vi "SerialCharWriteReadnoopen.vi"(0 "VISA resource name":refnum<visa-resource-name>, 3 "write buffer":string) -> (10 "read buffer":string)   [LabVIEW 2012]
doc: "The Basic Serial Read and Write example performs a Serial Port Read, a Serial Port Write, or a combination of these actions. The user selects the actions (read or write) on the front panel. If both are selected, the VI will write the data first, read data, and then close the VISA session that is opened to the port. This VI will wait until the specified number of bytes is received at the port. Only the number of bytes specified will be read.\n\nINSTRUCTIONS:\n1) Select the serial resource and configuration parameters (baud rate, data bits, parity, stop bits, flow control).\n2) Select the operations to be performed. \n3) Connect the serial port to your device. If no device is available, perform a loopback test by doing one of the following. Short pins 2 and 3 on a RS-232 cable or short pin 4 to pin 8 and pin 5 to pin 9 on a RS-485/422 cable. \n4) Run the VI to see the data read. (The \"read string\" will match the \"string to write\" if a loopback test was performed.)\n\nNote: The parameters set for the serial port must match the parameters of the connected instrument or device. In this example, the bytes to read parameter specifies the number of bytes that the serial port reads. If there were more bytes at the port than the number specified in bytes to read, those bytes would not be read. Also, if you specify to read more bytes than the number of bytes actually read, you might receive a timeout error message.\n\nOn the block diagram, the Configure Serial Port VI sets the configuration parameters. The front panel displays the controls used to configure the basic parameters, such as baud rate, data bits, and parity. Constants configure the other parameters the user probably does not need set. After the VISA Configure Serial Port VI opens the VISA session and configures the port, the VI passes the VISA resource name to other VIs that perform operations on that VISA resource. The VISA Write function sends a command to the serial device and the VISA Read function returns data based on the command. The VISA Close function then closes the reference to the serial device. It is important to close the reference; otherwise communication through with that port through protocols other than VISA might not be possible."
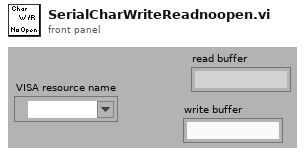
[diagram p1: front panel]
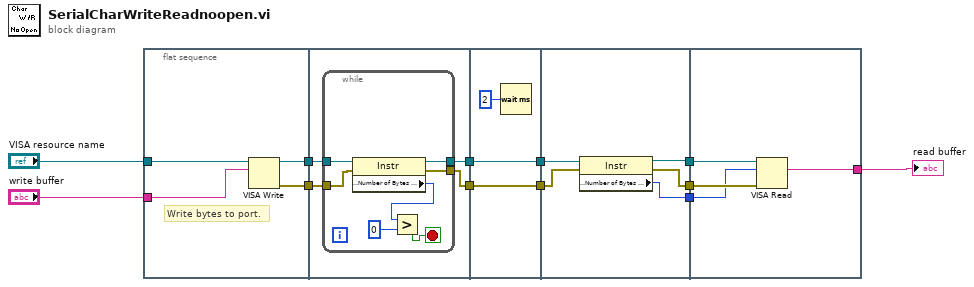
[diagram p0: block diagram]
diagram:
  n1 = flat-sequence {
    tunnel: "VISA resource name" -> [w16]
    tunnel: [w15] -> w7
    tunnel: [w14] -> w5
    tunnel: "write buffer" -> [w13]
    tunnel: w7 -> [w20]
    tunnel: [w19] -> w6
    tunnel: w5 -> [w18]
    tunnel: [w17] -> w4
    tunnel: w6 -> [w30]
    tunnel: w4 -> [w29]
    tunnel: [w30] -> w12
    tunnel: [w29] -> w10
    tunnel: w12 -> [w35]
    tunnel: [w34] -> w11
    tunnel: w10 -> [w33]
    tunnel: [w32] -> w9
    tunnel: [w31] -> w8
    tunnel: w11 -> [w39]
    tunnel: w9 -> [w38]
    tunnel: w8 -> [w37]
    tunnel: [w36] -> w2
    frame #0 {
      # "Write bytes to port."
      n2 = VISA Write(VISA resource name=w16, write buffer=w13) -> (VISA resource name out=w15:refnum<visa-resource-name>, error out=w14:errorcluster)  [unwired: 1 in, 1 out]
    }
    frame #1 {
      n3 = while {
        tunnel: w20 -> [w27]
        tunnel: [w26] -> w19
        tunnel: w18 -> [w25]
        tunnel: [w24] -> w17
        stop <- w21 stop-if-true
        n4 = property class="Instr"(reference=w27, error in=w25) -> (reference out=w26:refnum<visa-resource-name>, error out=w24:errorcluster, "Serial Settings:Number of Bytes at Serial Port"=w23:u32)
        n5 = Greater?(x=w23, y=u32 0) -> (0:w21:bool)
      }
    }
    frame #2 {
      n6 = Wait (ms)(milliseconds to wait=u32 2) -> ()  [unwired: 1 out]
    }
    frame #3 {
      n7 = property class="Instr"(reference=w35, error in=w33) -> (reference out=w34:refnum<visa-resource-name>, error out=w32:errorcluster, "Serial Settings:Number of Bytes at Serial Port"=w31:u32)
    }
    frame #4 {
      n8 = VISA Read(VISA resource name=w39, byte count=w37, error in (no error)=w38) -> (read buffer=w36:string)  [unwired: 3 out]
    }
  }
  "read buffer" <- w2
